vi "unflattenPressureFromXML_Scalar.vi"(8 "error in (no error)":errorcluster, 9 "pressureUnitInXML":T1, 10 "xmlString":string, 11 "pressureForType":dbl[unit]) -> (0 "error out":errorcluster, 3 "pressure":dbl[unit])   [LabVIEW 2016, in "UnitsAndXML.lvlib"]
uses:
  <userlib>/Common/UnitsAndXML/UnitsAndXML.lvlib
  <userlib>/Common/UnitsAndXML/FlattenItemWithUnitToXML/FlattenPressureToXML/PressureUnit.ctl
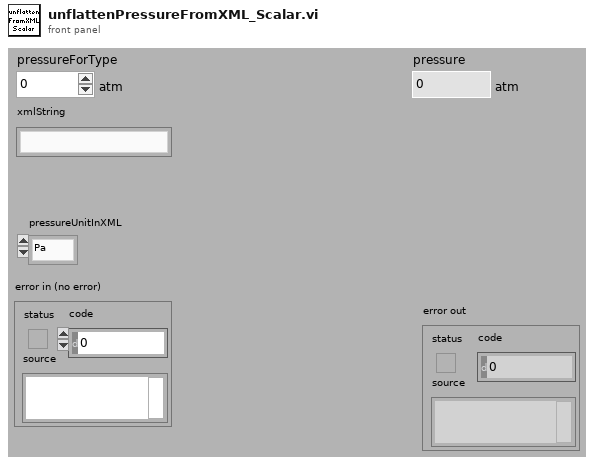
[diagram p1: front panel]
types:
  T1 = typedef "UnitsAndXML.lvlib/PressureUnit.ctl" = enum16{"Pa", "atm", "bar", "mbar", "m.Hg", "psi", "torr"}
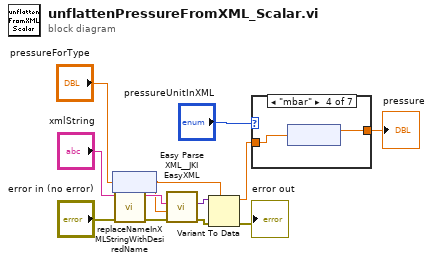
[diagram p0: block diagram]
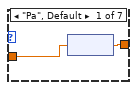
[diagram p2: hidden frame]
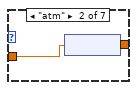
[diagram p3: hidden frame]
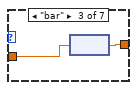
[diagram p4: hidden frame]
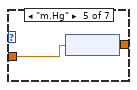
[diagram p5: hidden frame]
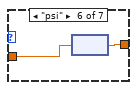
[diagram p6: hidden frame]
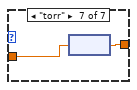
[diagram p7: hidden frame]
diagram:
  n1 = node("pressureForType") -> (w7:dbl)
  n2 = call <userlib>:"replaceNameInXMLStringWithDesiredName.vi"("error in"="error in (no error)", "xmlString"="xmlString") -> ("error out"=w1:errorcluster, "revisedXMLString"=w9:string)  [unwired: 8 in]
  n3 = call <vilib>:"Easy Parse XML__JKI EasyXML.vi"("error in (no error)"=w1, "LabVIEW Data (Type)"=w7, "XML String"=w9) -> ("error out"=w4:errorcluster, "LabVIEW Data"=w11:variant)  [unwired: 7 in]
  n4 = Variant To Data(error in=w4, type=w7, Variant=w11) -> (data=w6:dbl, error out=→"error out":errorcluster)
  n5 = case shown="\"mbar\"" "pressureUnitInXML" {
    tunnel: w6 -> [w14 w16 w18 w20 w22 w24 w26]
    tunnel: [w13 w15 w17 w19 w21 w23 w25] -> w5
    frame "Pa", Default {
      n6 = node(w14) -> (w13:dbl[unit])
    }
    frame "atm" {
      n7 = node(w16) -> (w15:dbl[unit])
    }
    frame "bar" {
      n8 = node(w18) -> (w17:dbl[unit])
    }
    frame "mbar" {
      n9 = node(w20) -> (w19:dbl[unit])
    }
    frame "m.Hg" {
      n10 = node(w22) -> (w21:dbl[unit])
    }
    frame "psi" {
      n11 = node(w24) -> (w23:dbl[unit])
    }
    frame "torr" {
      n12 = node(w26) -> (w25:dbl[unit])
    }
  }
  "pressure" <- w5
